vi "GOOPUtil_FindObjectAttributesFolderPath.vi"(0 "application reference (local)":refnum<vi>, 2 "GOOPKernelName":string, 5 "error in (no error)":errorcluster) -> (15 "Folder":path, 19 "error out":errorcluster)   [LabVIEW 2014, in "GOOPUtility.lvlib"]
doc: "Finds the objects attribute path from the GOOPKernel full VI name."
uses:
  <vilib>/addons/GOOPUtility/GOOPUtility.lvlib
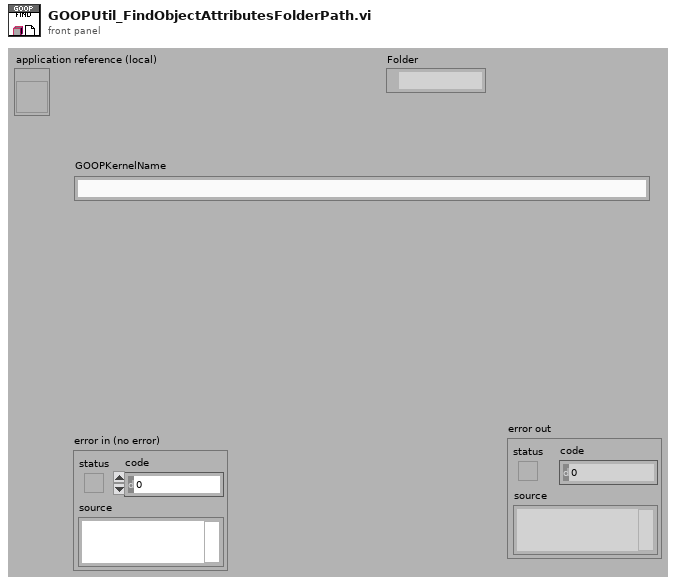
[diagram p1: front panel]
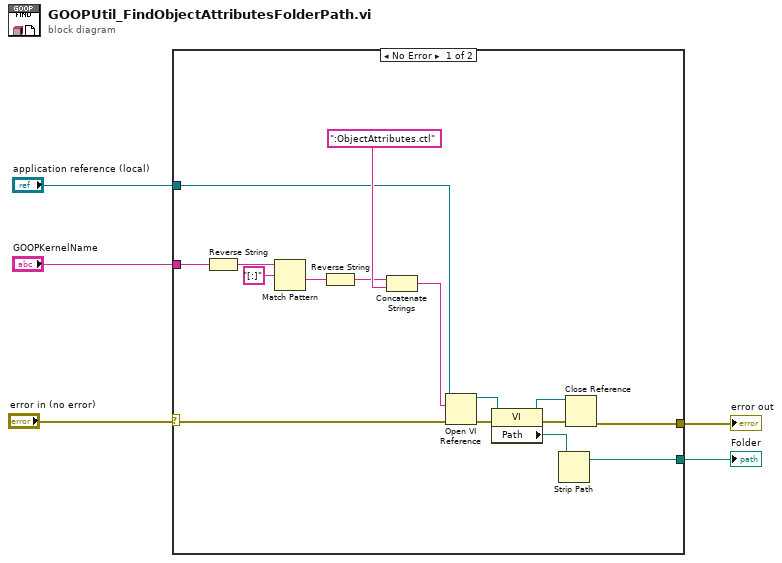
[diagram p0: block diagram]
diagram:
  n1 = case shown="No Error" "error in (no error)" {
    selector: "error in (no error)" -> [w12 w22]
    tunnel: "GOOPKernelName" -> [w11 _]
    tunnel: "application reference (local)" -> [w6 _]
    tunnel: [w14 w22] -> w3
    tunnel: [w13 _] -> w2
    frame No Error {
      n2 = Reverse String(1:w11) -> (0:w9:string)
      n3 = Match Pattern(string=w9, regular expression="[:]") -> (after substring=w8:string)  [unwired: 1 in, 3 out]
      n4 = Reverse String(1:w8) -> (0:w7:string)
      n5 = Concatenate Strings(w7, ":ObjectAttributes.ctl") -> (w15:string)
      n6 = Open VI Reference(application reference (local)=w6, vi path=w15, error in (no error)=w12) -> (vi reference=w20:refnum<vi>, error out=w21:errorcluster)  [unwired: 3 in]
      n7 = property class="VI"(reference=w20, error in=w21) -> (reference out=w18:refnum<vi>, error out=w19:errorcluster, "Path"=w17:path)
      n8 = Strip Path(path=w17) -> (stripped path=w13:path)  [unwired: 1 out]
      n9 = Close Reference(reference=w18, error in (no error)=w19) -> (error out=w14:errorcluster)
    }
    frame Error {
    }
  }
  "error out" <- w3
  "Folder" <- w2
